vi "报文拆分.vi"(0 "报文":string) -> (16 "拆分报告":T1)   [LabVIEW 2019, in "MainPage.lvlib" / "MainPage.lvclass"]
uses:
  MainPage.lvclass
panel:
  in  "报告模板":T1
  # "规定输出格式：\n原报文\n判定分类\n属性拆分\n  通讯地址\n  功能码\n  功能属性1\n  功能属性2\n  数据"
  # "都是字符串方便后续整合"
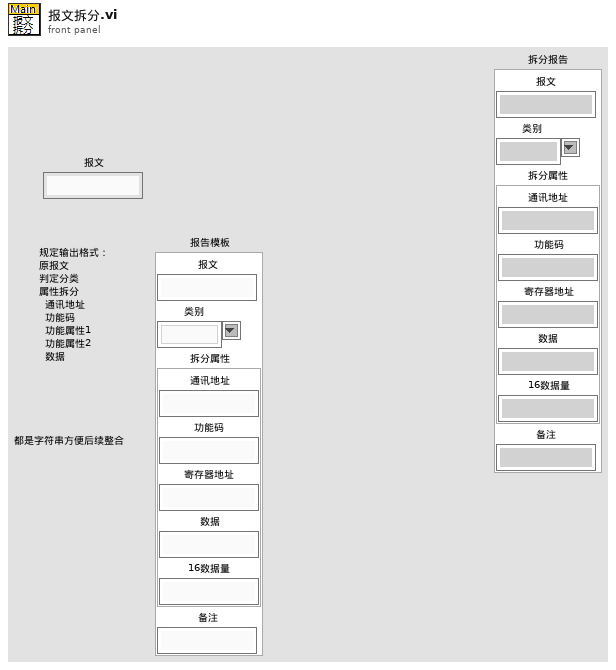
[diagram p1: front panel]
types:
  T1 = cluster{"报文":string, "类别":string, "拆分属性":cluster{"通讯地址":string, "功能码":string, "寄存器地址":string, "数据":string, "16数据量":string}, "备注":string}
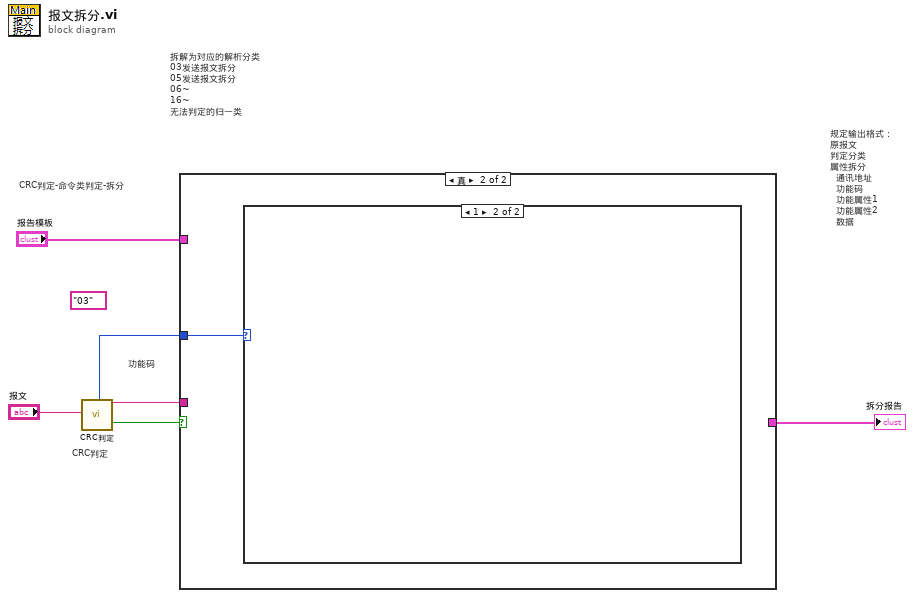
[diagram p0: block diagram]
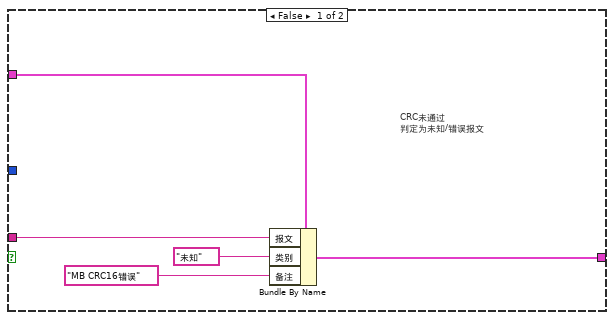
[diagram p2: hidden frame]
diagram:
  (unwired) "03" ("类别")
  # "功能码"
  # "规定输出格式：\n原报文\n判定分类\n属性拆分\n  通讯地址\n  功能码\n  功能属性1\n  功能属性2\n  数据"
  # "CRC判定"
  # "CRC判定-命令类判定-拆分"
  # "拆解为对应的解析分类\n03发送报文拆分\n05发送报文拆分\n06~\n16~\n无法判定的归一类"
  n1 = call "CRC判定.vi"("报文"="报文") -> ("功能码"=w1:u8, "报文输出"=w4:string, "CRC正确"=w5:bool)  [unwired: 16 in]
  n2 = case shown="真" w5 {
    tunnel: w4 -> [w10 _]
    tunnel: "报告模板" -> [w11 _]
    tunnel: [w8 _] -> w2
    tunnel: w1 -> [_ w12]
    frame False {
      # "CRC未通过\n判定为未知/错误报文"
      n3 = Bundle By Name(cluster=w11, "报文"=w10, "类别"="未知", "备注"="MB CRC16错误") -> (w8:T1)
    }
    frame True {
      n4 = case shown="1" w12 {
        frame 0, Default {
        }
        frame 1 {
        }
      }
    }
  }
  "拆分报告" <- w2
